vi "Global 1.vi"() -> ()   [LabVIEW 2015]
panel:
  in  "Stop":bool
  in  "Voltage_measurements":dbl
  in  "x":dbl
  in  "current_measurements":dbl
  in  "i":dbl
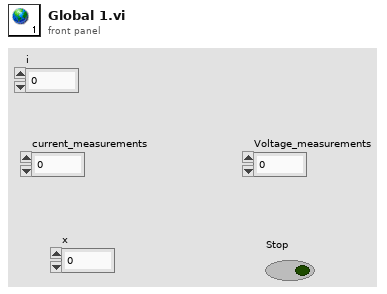
[diagram p1: front panel]
diagram:
